vi "GetConfiguration.vi"(8 "error in":errorcluster) -> (0 "error out":errorcluster, 2 "cancelled":bool, 3 "Cluster":T1)   [LabVIEW 2013]
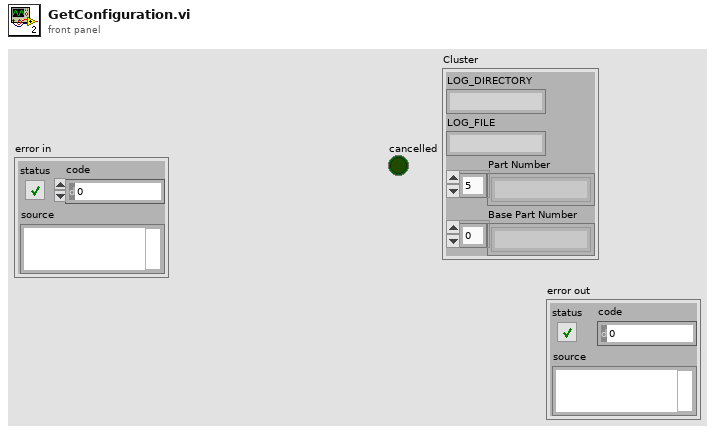
[diagram p1: front panel]
types:
  T1 = cluster{"LOG_DIRECTORY":string, "LOG_FILE":string, "Part Number":string[], "Base Part Number":string[]}
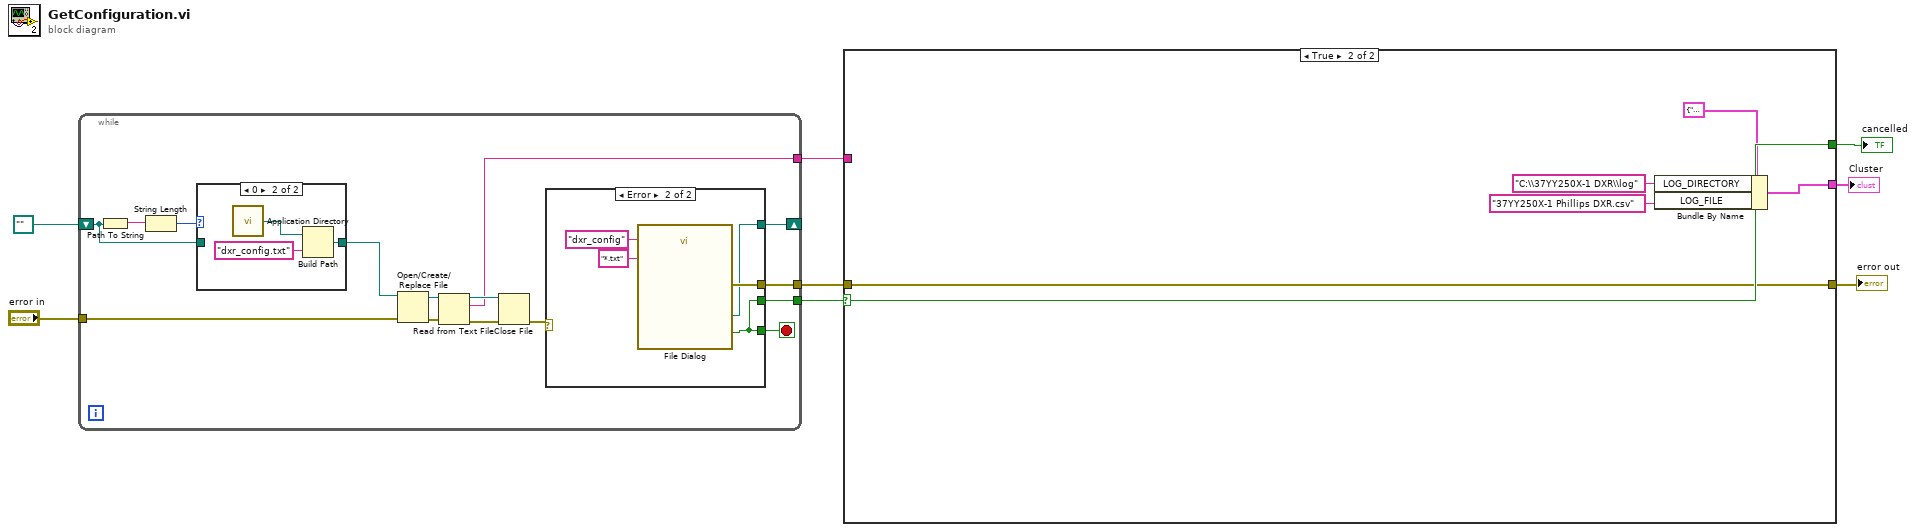
[diagram p0: block diagram]
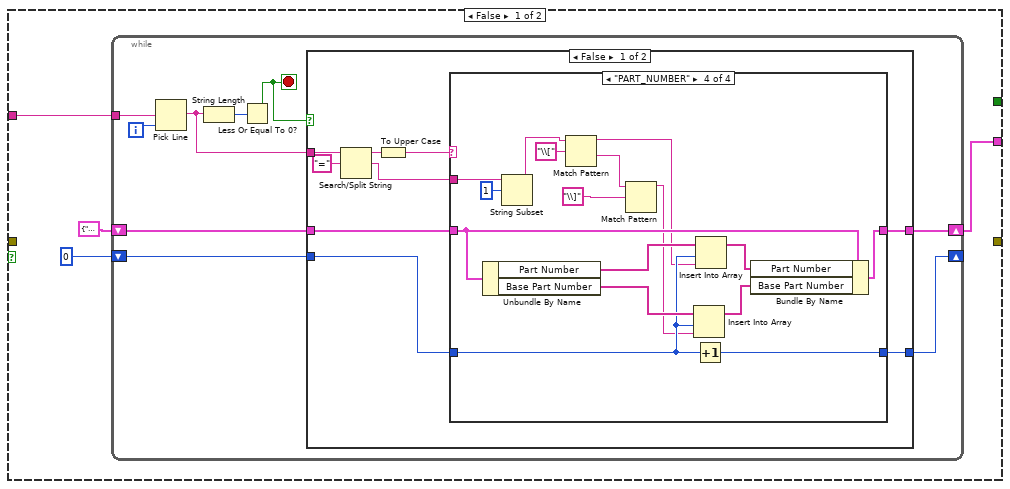
[diagram p2: hidden frame]
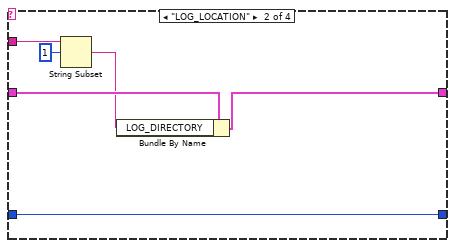
[diagram p4: hidden frame]
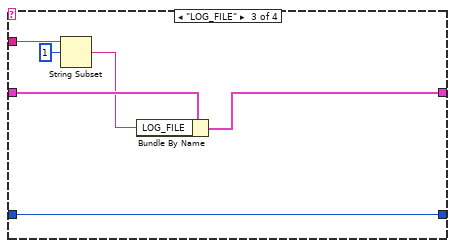
[diagram p5: hidden frame]
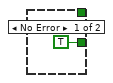
[diagram p8: hidden frame]
diagram:
  n1 = while {
    tunnel: [w18] -> w8
    tunnel: "error in" -> [w17]
    tunnel: [w15] -> w3
    shift-right: [w13] -> _
    shift-left: path "" ("selected path") -> [w9]
    tunnel: [w12] -> w6
    stop <- w14 stop-if-true
    n2 = Path To String(path=w9) -> (string=w11:string)
    n3 = String Length(string=w11) -> (length=w10:i32)
    n4 = case shown="0" w10 {
      tunnel: [w24 w26] -> w19
      tunnel: w9 -> [w24 _]
      frame 1, Default {
      }
      frame 0 {
        n5 = call <vilib>:"Application Directory.vi"() -> ("Application Directory"=w27:path)
        n6 = Build Path(base path=w27, name or relative path="dxr_config.txt") -> (appended path=w26:path)
      }
    }
    n7 = Open/Create/Replace File(file path (use dialog)=w19, error in=w17) -> (refnum out=w22:refnum<file>, error out=w23:errorcluster)  [unwired: 4 in, 1 out]
    n8 = Read from Text File(file (use dialog)=w22, error in=w23) -> (refnum out=w20:refnum<file>, text=w18:string, error out=w21:errorcluster)  [unwired: 2 in, 1 out]
    n9 = Close File(refnum=w20, error in=w21) -> (error out=w16:errorcluster)  [unwired: 1 out]
    n10 = case shown="Error" w16 {
      tunnel: [_ w31] -> w15
      tunnel: [TRUE ("cancelled") w29] -> w14
      tunnel: [_ w30] -> w13
      tunnel: [_ w29] -> w12
      frame No Error {
      }
      frame Error {
        n11 = call "File Dialog"("default name"="dxr_config", "pattern (all files)"="*.txt") -> ("selected path"=w30:path, "cancelled"=w29:bool, "error out"=w31:errorcluster)  [unwired: 10 in, 1 out]
      }
    }
  }
  n12 = case shown="True" w6 {
    selector: w6 -> [_ w93]
    tunnel: [w37 w90] -> w1
    tunnel: w8 -> [w36 _]
    tunnel: [_ w93] -> w5
    tunnel: [_ w92] -> w4
    tunnel: w3 -> [_ w92]
    frame False {
      n13 = while {
        tunnel: w36 -> [w46]
        shift-right: [w40] -> w37
        shift-left: T1 {"LOG_DIRECTORY"="", "LOG_FILE"="", "Part Number"=[], "Base Part Number"=[]} ("Cluster") -> [w42]
        shift-right: [w38] -> _
        shift-left: 0 -> [w39]
        i -> [w45]
        stop <- w43 stop-if-true
        n14 = Pick Line(multi-line string=w46, line index=w45) -> (output string=w41:string)  [unwired: 1 in]
        n15 = String Length(string=w41) -> (length=w44:i32)
        n16 = Less Or Equal To 0?(x=w44) -> (x <= 0?=w43:bool)
        n17 = case shown="False" w43 {
          tunnel: w42 -> [w50 w87]
          tunnel: w41 -> [w55 _]
          tunnel: [w49 w87] -> w40
          tunnel: w39 -> [w48 w86]
          tunnel: [w47 w86] -> w38
          frame False {
            n18 = Search/Split String(string=w55, search string/char (-)="=") -> (substring before match=w52:string, match + rest of string=w51:string)  [unwired: 1 in, 1 out]
            n19 = To Upper Case(1:w52) -> (0:w53:string)
            n20 = case shown="\"PART_NUMBER\"" w53 {
              tunnel: w51 -> [_ w63 w69 w85]
              tunnel: w50 -> [w57 w61 w67 w83]
              tunnel: [w57 w60 w66 w82] -> w49
              tunnel: w48 -> [w56 w58 w64 w76]
              tunnel: [w56 w58 w64 w77] -> w47
              frame "False", Default {
              }
              frame "LOG_LOCATION" {
                n21 = String Subset(string=w63, offset (0)=1) -> (substring=w59:string)  [unwired: 1 in]
                n22 = Bundle By Name(cluster=w61, "LOG_DIRECTORY"=w59) -> (w60:T1)
              }
              frame "LOG_FILE" {
                n23 = String Subset(string=w69, offset (0)=1) -> (substring=w65:string)  [unwired: 1 in]
                n24 = Bundle By Name(cluster=w67, "LOG_FILE"=w65) -> (w66:T1)
              }
              frame "PART_NUMBER" {
                n25 = Unbundle By Name(w83) -> ("Part Number"=w81:string[], "Base Part Number"=w80:string[])
                n26 = String Subset(string=w85, offset (0)=1) -> (substring=w72:string)  [unwired: 1 in]
                n27 = Match Pattern(string=w72, regular expression="\\[") -> (before substring=w70:string, after substring=w74:string)  [unwired: 1 in, 2 out]
                n28 = Match Pattern(string=w74, regular expression="\\]") -> (before substring=w71:string)  [unwired: 1 in, 3 out]
                n29 = Insert Into Array(array=w80, index=w76, new element=w71) -> (w79:string[])
                n30 = Increment(x=w76) -> (x+1=w77:i32)
                n31 = Insert Into Array(array=w81, index=w76, new element=w70) -> (w78:string[])
                n32 = Bundle By Name(cluster=w83, "Part Number"=w78, "Base Part Number"=w79) -> (w82:T1)
              }
            }
          }
          frame True {
          }
        }
      }
    }
    frame True {
      n33 = Bundle By Name(cluster=T1 {"LOG_DIRECTORY"="", "LOG_FILE"="", "Part Number"=[], "Base Part Number"=[]} ("Cluster 2"), "LOG_DIRECTORY"="C:\\37YY250X-1 DXR\\log", "LOG_FILE"="37YY250X-1 Phillips DXR.csv") -> (w90:T1)
    }
  }
  "error out" <- w4
  "cancelled" <- w5
  "Cluster" <- w1
